vi "Add Async Message to Map.vi"(8 "error in (no error)":errorcluster, 10 "Message":refnum<class "Async Message.lvclass">, 11 "Async Methods Actor in":refnum<class "Async Methods Actor.lvclass">) -> (0 "error out":errorcluster, 3 "Async Methods Actor out":refnum<class "Async Methods Actor.lvclass">)   [LabVIEW 2023, in "Async Methods Actor.lvlib" / "Async Methods Actor.lvclass"]
uses:
  Async Methods Actor.lvclass
  Async Methods Actor Messages/Async Message/Async Message.lvclass
  Async Methods Actor.lvclass/Async Methods Actor.ctl
  Async Methods Actor Messages/Async Message/Async Message.lvclass/Async Message.ctl
  Async Message Execution Status.ctl
  Write Async Message Execution Status Map.vi
  Async Methods Actor Messages/Async Message/Read FQN.vi
  Async Methods Actor Messages/Async Message/Read Async Call Method.vi
  Write Async Message Execution Status Map.vi/3adbf29e-89d7-4ecb-a2bd-8a8b89d527f8.vi
  Get VI FQN.vi
  <vilib>/Utility/LVClass/Get LV Class Path.vi
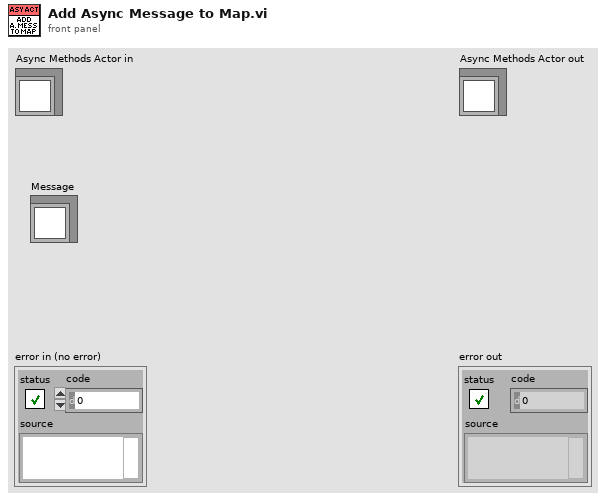
[diagram p1: front panel]
types:
  T1 = typedef "Async Methods Actor.lvlib/Async Methods Actor.lvclass/Async Message Execution Status.ctl" = cluster{"C&C Clones Running":u32, "C&F Clones Launched":u32}
  T2 = typedef "Async Methods Actor.lvlib/Async Methods Actor.lvclass/Async Call Method.ctl" = enum16{"Call and Collect", "Call and Forget"}
  T3 = typedef "Async Methods Actor.lvlib/Async Methods Actor.lvclass/Async Message Execution Status Map.ctl" = map{string, T1}
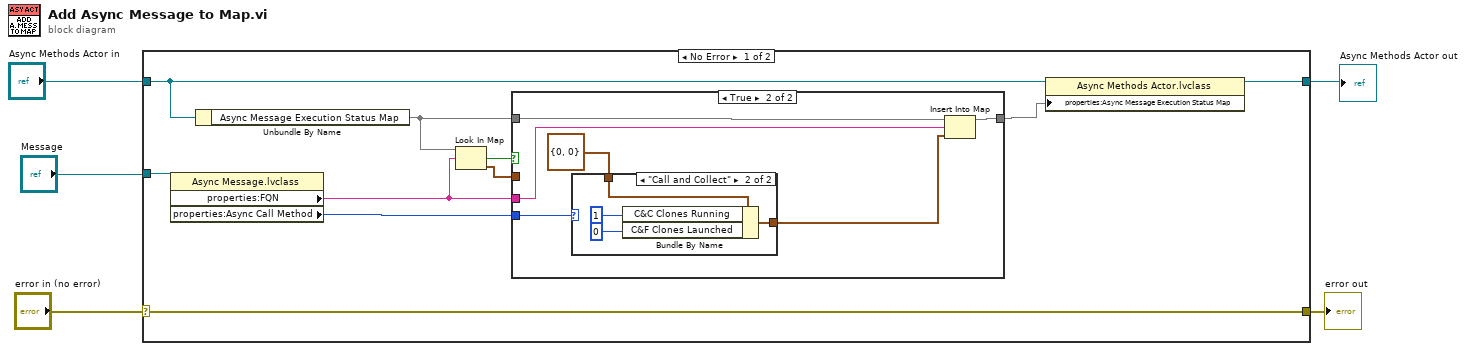
[diagram p0: block diagram]
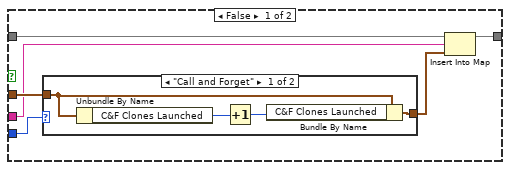
[diagram p2: hidden frame]
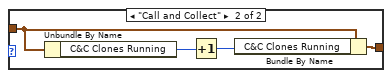
[diagram p3: hidden frame]
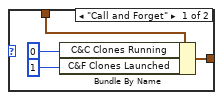
[diagram p4: hidden frame]
diagram:
  n1 = case shown="No Error" "error in (no error)" {
    selector: "error in (no error)" -> [w15 w45]
    tunnel: [w15 w45] -> w4
    tunnel: [w9 w44] -> w2
    tunnel: "Async Methods Actor in" -> [w10 w44]
    tunnel: "Message" -> [w8 _]
    frame No Error {
      n2 = property class="Async Message.lvclass"(reference=w8) -> ("properties:FQN"=w7:string, "properties:Async Call Method"=w6:T2)  [unwired: 1 in, 2 out]
      n3 = Unbundle By Name(w10) -> ("Async Message Execution Status Map"=w14:T3)
      n4 = Look In Map(map=w14, key=w7) -> (key not found?=w13:bool, value=w12:T1)  [unwired: 1 in]
      n5 = case shown="True" w13 {
        tunnel: w7 -> [w18 w35]
        tunnel: w14 -> [w19 w34]
        tunnel: w12 -> [w20 _]
        tunnel: w6 -> [w16 w31]
        tunnel: [w21 w32] -> w11
        frame False {
          n6 = case shown="\"Call and Forget\"" w16 {
            tunnel: w20 -> [w24 w28]
            tunnel: [w22 w26] -> w17
            frame "Call and Forget" {
              n7 = Unbundle By Name(w24) -> ("C&F Clones Launched"=w25:u32)
              n8 = Increment(x=w25) -> (x+1=w23:u32)
              n9 = Bundle By Name(cluster=w24, "C&F Clones Launched"=w23) -> (w22:T1)
            }
            frame "Call and Collect" {
              n10 = Unbundle By Name(w28) -> ("C&C Clones Running"=w29:u32)
              n11 = Increment(x=w29) -> (x+1=w27:u32)
              n12 = Bundle By Name(cluster=w28, "C&C Clones Running"=w27) -> (w26:T1)
            }
          }
          n13 = Insert Into Map(map in=w19, key=w18, value=w17) -> (map out=w21:T3)  [unwired: 2 out]
        }
        frame True {
          n14 = case shown="\"Call and Collect\"" w31 {
            tunnel: [w38 w42] -> w33
            tunnel: T1 {"C&C Clones Running"=0, "C&F Clones Launched"=0} ("value") -> [w36 w40]
            frame "Call and Forget" {
              n15 = Bundle By Name(cluster=w36, "C&C Clones Running"=u32 0, "C&F Clones Launched"=u32 1 ("Number of Clones")) -> (w38:T1)
            }
            frame "Call and Collect" {
              n16 = Bundle By Name(cluster=w40, "C&C Clones Running"=u32 1, "C&F Clones Launched"=u32 0 ("Number of Clones")) -> (w42:T1)
            }
          }
          n17 = Insert Into Map(map in=w34, key=w35, value=w33) -> (map out=w32:T3)  [unwired: 2 out]
        }
      }
      n18 = property class="Async Methods Actor.lvclass"(reference=w10, "properties:Async Message Execution Status Map"=w11) -> (reference out=w9:refnum<class "Async Methods Actor.lvclass">)  [unwired: 1 in, 1 out]
    }
    frame Error {
    }
  }
  "error out" <- w4
  "Async Methods Actor out" <- w2
